vi "Get XYZ dimensions for VL patches.vi"(8 "error in (no error)":errorcluster, 10 "Stop coordinates":T2, 11 "Start coordinates":T1) -> (0 "error out":errorcluster, 1 "DeltaZ":i32, 2 "DeltaY":i32, 3 "DeltaX":i32, 4 "Single Plane ROI":bool, 5 "X < Y?":bool)   [LabVIEW 2020]
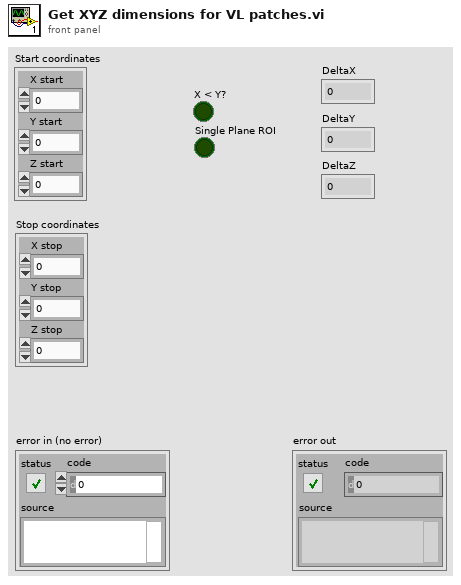
[diagram p1: front panel]
types:
  T1 = cluster{"X start":i32, "Y start":i32, "Z start":i32}
  T2 = cluster{"X stop":i32, "Y stop":i32, "Z stop":i32}
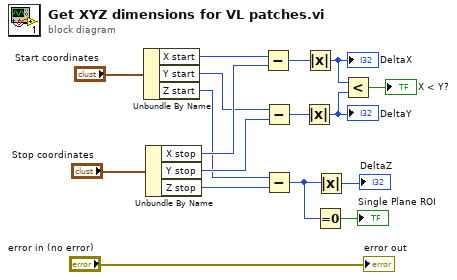
[diagram p0: block diagram]
diagram:
  n1 = Unbundle By Name("Start coordinates") -> ("X start"=w15:i32, "Y start"=w13:i32, "Z start"=w11:i32)
  n2 = Unbundle By Name("Stop coordinates") -> ("X stop"=w14:i32, "Y stop"=w12:i32, "Z stop"=w10:i32)
  n3 = Subtract(x=w15, y=w14) -> (x-y=w7:i32)
  n4 = Subtract(x=w13, y=w12) -> (x-y=w6:i32)
  n5 = Subtract(x=w11, y=w10) -> (x-y=w4:i32)
  n6 = Absolute Value(x=w6) -> (abs(x)=w1:i32)
  "DeltaY" <- w1
  n7 = Absolute Value(x=w7) -> (abs(x)=w2:i32)
  "DeltaX" <- w2
  n8 = Equal To 0?(x=w4) -> (x = 0?=→"Single Plane ROI":bool)
  n9 = Absolute Value(x=w4) -> (abs(x)=→"DeltaZ":i32)
  n10 = Less?(x=w2, y=w1) -> (x < y?=→"X < Y?":bool)
  "error out" <- "error in (no error)"
